vi "Init Remote Services.vi"(8 "error in (no error)":errorcluster, 11 "Vecto in":refnum<class "Vecto.lvclass">) -> (0 "error out":errorcluster, 3 "Vecto out":refnum<class "Vecto.lvclass">)   [LabVIEW 2020, in "Vecto.lvlib" / "Vecto.lvclass"]
uses:
  Vecto.lvclass
  Vecto.lvclass/Vecto.ctl
  Event Level.ctl
  Vecto.lvlib
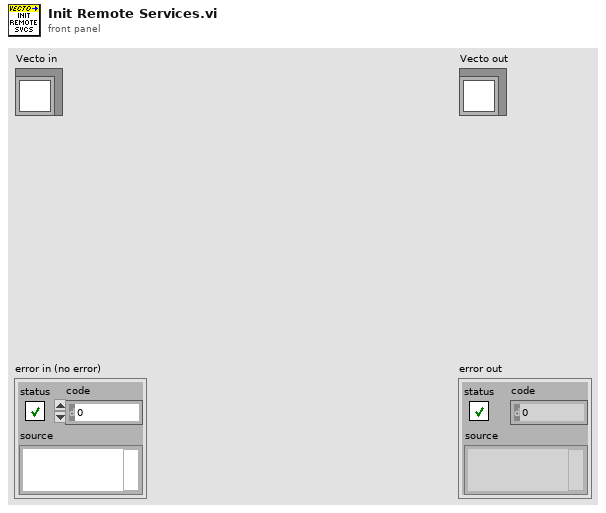
[diagram p1: front panel]
types:
  T1 = typedef "Vecto.lvlib/Event Level.ctl" = enum16{"Debug", "Info", "Warning", "Error"}
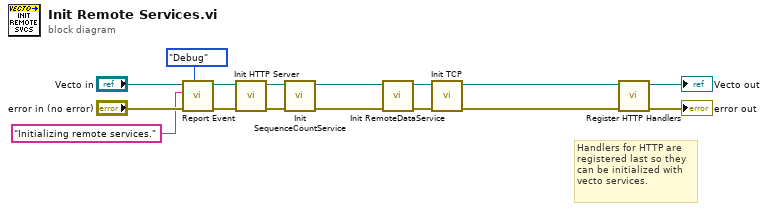
[diagram p0: block diagram]
diagram:
  # "Handlers for HTTP are registered last so they can be initialized with vecto services."
  n1 = call "Report Event.vi"("Event Level (Info)"=Event_Level."Debug", "error in (no error)"="error in (no error)", "Message"="Initializing remote services.", "Vecto in"="Vecto in") -> ("error out"=w7:errorcluster, "Vecto out"=w5:refnum<class "Vecto.lvclass">)  [unwired: 6 in]
  n2 = call "Init HTTP Server.vi"("error in (no error)"=w7, "Vecto in"=w5) -> ("error out"=w14:errorcluster, "Vecto out"=w13:refnum<class "Vecto.lvclass">)  [unwired: 8 in]
  n3 = call "Init SequenceCountService.vi"("error in (no error)"=w14, "Vecto in"=w13) -> ("error out"=w1:errorcluster, "Vecto out"=w2:refnum<class "Vecto.lvclass">)  [unwired: 8 in]
  n4 = call "Init RemoteDataService.vi"("error in (no error)"=w1, "Vecto in"=w2) -> ("error out"=w15:errorcluster, "Vecto out"=w9:refnum<class "Vecto.lvclass">)  [unwired: 8 in]
  n5 = call "Init TCP.vi"("error in (no error)"=w15, "Vecto in"=w9) -> ("error out"=w10:errorcluster, "Vecto out"=w8:refnum<class "Vecto.lvclass">)  [unwired: 8 in]
  n6 = call "Register HTTP Handlers.vi"("error in (no error)"=w10, "Vecto in"=w8) -> ("error out"=→"error out":errorcluster, "Vecto out"=→"Vecto out":refnum<class "Vecto.lvclass">)  [unwired: 8 in]
